vi "lecture_grating.vi"(11 "GratingSelected":string) -> (3 "array":string[](array[string]))   [LabVIEW 2019]
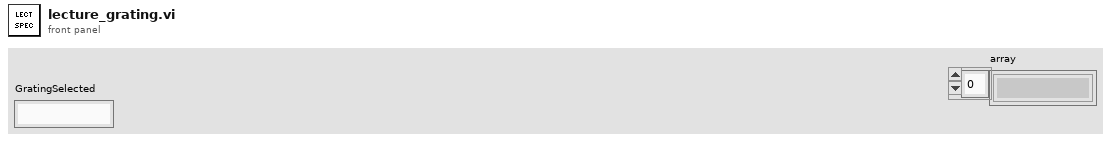
[diagram p1: front panel]
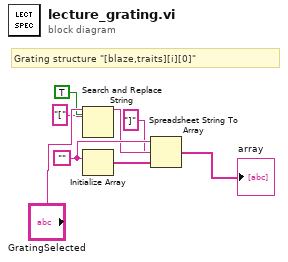
[diagram p0: block diagram]
diagram:
  w5 = "" ("format string")
  # "Grating structure \"[blaze,traits][i][0]\""
  n1 = Search and Replace String(replace all?=TRUE, input string="GratingSelected", search string="[") -> (result string=w4:string)  [unwired: 5 in, 3 out]
  n2 = Initialize Array(w5) -> (w6:string[])  [unwired: 1 in]
  n3 = Spreadsheet String To Array(delimiter (Tab)="]", format string=w5, spreadsheet string=w4, array type (2D Dbl)=w6) -> (array=→"array":string[])
